vi "Signal_Output.vi"(8 "Fs (Hz)":dbl=1000.0, 9 "Stop":bool, 10 "Waveform settings":T1={"Vx_max"=0.3, "Vy_max"=1.0, "T"=1.0, "Row_N"=20, "ratio of decline"=0.3}) -> (0 "Y":waveform(dbl)(graph), 1 "X":waveform(dbl)(graph), 3 "XY图":cluster{"X":dbl, "Y":dbl}[](graph))   [LabVIEW 2013]
panel:
  out "滑动杆":u32(slide) scale=0.0..1536000000.0
  # "Tx: x方向每行扫描时间\nVx_max: x方向最大电压幅值\nVy_max: y方向最大电压幅值\nRowN: 扫描行数\nratio of decline: 每行卷回时间占每行扫描时间的比例\nFs: frequency of sampling"
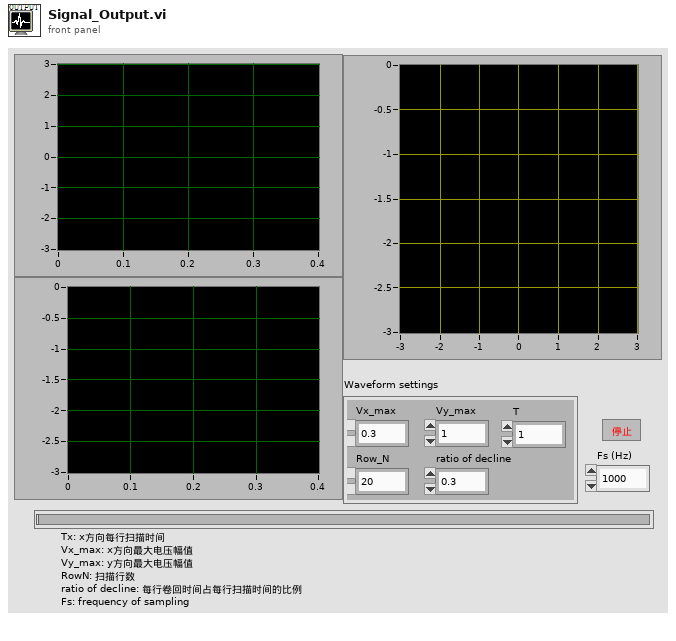
[diagram p1: front panel]
types:
  T1 = cluster{"Vx_max":dbl, "Vy_max":dbl, "T":dbl, "Row_N":i32, "ratio of decline":dbl}
  T2 = cluster{"T":dbl, "Vx_max":dbl, "Vy_max":dbl, "Row_N":i32, "ratio of decline":dbl, dbl}
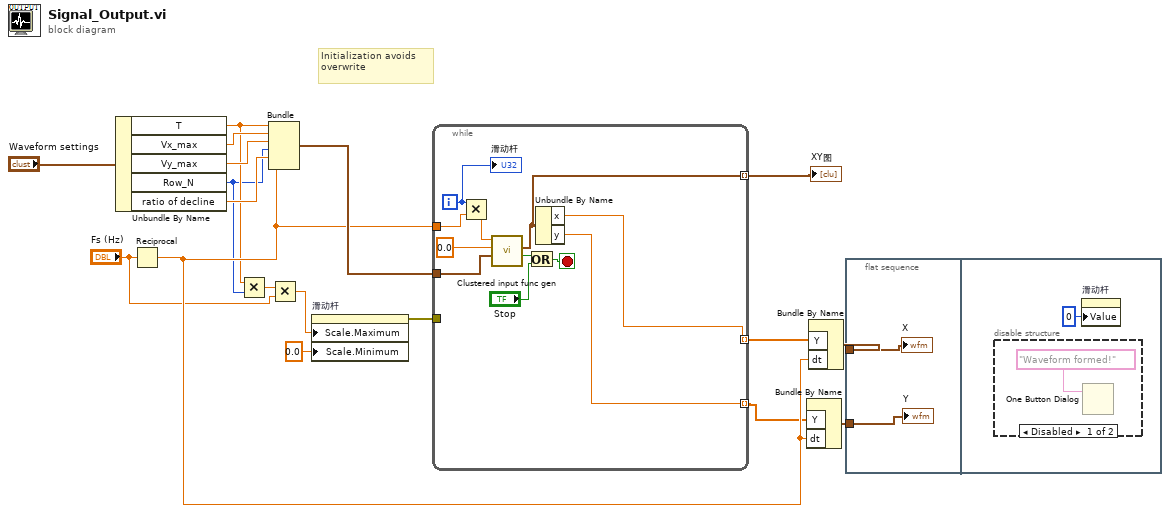
[diagram p0: block diagram]
diagram:
  # "Initialization avoids\noverwrite"
  n1 = Unbundle By Name("Waveform settings") -> ("T"=w6:dbl, "Vx_max"=w16:dbl, "Vy_max"=w15:dbl, "Row_N"=w5:i32, "ratio of decline"=w14:dbl)
  n2 = Reciprocal(x="Fs (Hz)") -> (1/x=w12:dbl)
  n3 = Multiply(x=w6, y=w5) -> (x*y=w4:dbl)
  n4 = Bundle("T"=w6, "Vx_max"=w16, "Vy_max"=w15, "Row_N"=w5, "ratio of decline"=w14, w12) -> (w13:T2)  [unwired: 1 in]
  n5 = Multiply(x=w4, y="Fs (Hz)") -> (x*y=w2:dbl)
  n6 = property on="滑动杆" class="Slide (严格)"("Scale.Maximum"=w2, "Scale.Minimum"=0.0 ("标尺.范围:最小值")) -> (error out=w7:errorcluster)  [unwired: 2 in, 1 out]
  n7 = while {
    tunnel: w13 -> [w26]
    tunnel: w12 -> [w24]
    tunnel: [w22] -> w11 mode=indexing
    tunnel: [w20] -> w10 mode=indexing
    tunnel: [w19] -> w9 mode=indexing
    tunnel: w7 -> [_]
    i -> [w21]
    stop <- w28 stop-if-true
    n8 = Multiply(x=w21, y=w24) -> (x*y=w23:dbl)
    n9 = call "Clustered input func gen.vi"("Settings"=w26, "beginning time"=0.0, "current time"=w23) -> ("finished?"=w27:bool, "x-y output"=w22:cluster{"x":dbl, "y":dbl})  [unwired: 6 in, 1 out]
    n10 = Or(x=w27, y="Stop") -> (x .or. y?=w28:bool)
    n11 = Unbundle By Name(w22) -> ("x"=w19:dbl, "y"=w20:dbl)
    "滑动杆" <- w21
  }
  "XY图" <- w11
  n12 = Bundle By Name("Y"=w10, "dt"=w12) -> (w17:waveform(dbl))  [unwired: 1 in]
  n13 = Bundle By Name("Y"=w9, "dt"=w12) -> (w18:waveform(dbl))  [unwired: 1 in]
  n14 = flat-sequence {
    tunnel: w18 -> [w31]
    tunnel: w17 -> [w30]
    frame #0 {
      "X" <- w31
      "Y" <- w30
    }
    frame #1 {
      n15 = disable-structure shown="Disabled" {
        frame Disabled {
          n16 = One Button Dialog(message="Waveform formed!" ("消息")) -> ()  [unwired: 1 in, 1 out]
        }
        frame Enabled {
        }
      }
      n17 = property on="滑动杆" class="Slide (严格)"("Value"=u32 0 ("滑动杆")) -> ()  [unwired: 2 in, 2 out]
    }
  }
